vi "Force Offset Tags DAO.vi"(8 "error in (no error)":errorcluster, 11 "DAO Actions":T1) -> (0 "error out":errorcluster, 2 "Force Tags":string[](array[string]))   [LabVIEW 2009]
uses:
  Data Access Objects/Metadata/DAO Actions.ctl
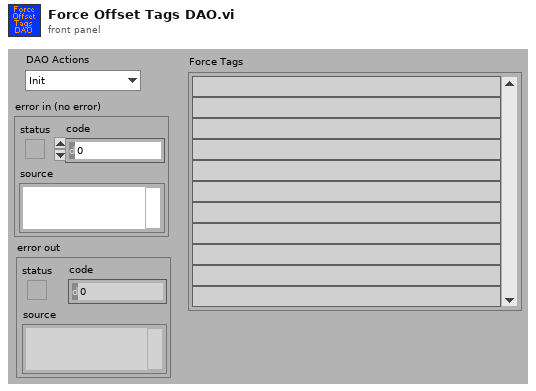
[diagram p1: front panel]
types:
  T1 = typedef "DAO Actions.ctl" = enum16{"Init", "Get", "Set"}
  T2 = typedef "Dataset Transaction Id.ctl" = cluster{"Dataset Source":T3, "Dataset Type":T4, "Hold":T5, "Volts":T5, "Tag":string}
  T3 = typedef "Dataset Source.ctl" = enum16{"LBCB 1", "LBCB 2", "Combined", "External Sensors"}
  T4 = typedef "Dataset Type.ctl" = enum16{"LVDT", "Load Cell", "Actuator Command", "Servo Error", "Displacement Command", "Displacement", "Force"}
  T5 = typedef "Yes No Button.ctl" = bool
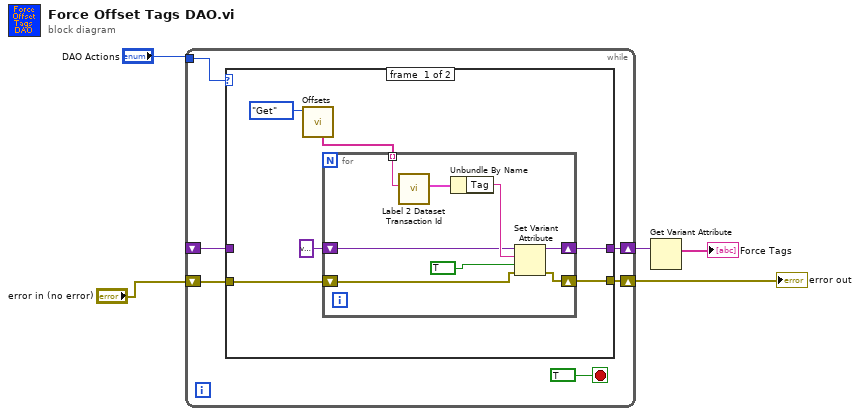
[diagram p0: block diagram]
diagram:
  n1 = while {
    tunnel: "DAO Actions" -> [w10]
    shift-right: [w9] -> w4
    shift-left: _ -> [w8]
    shift-right: [w6] -> w1
    shift-left: "error in (no error)" -> [w7]
    stop <- TRUE stop-if-true
    n2 = case shown="\"Init\", Default" w10 {
      tunnel: [w15 w27] -> w9
      tunnel: w8 -> [_ w27]
      tunnel: w7 -> [w13 w26]
      tunnel: [w12 w26] -> w6
      frame #0 {
        n3 = call "Offsets.vi"("DAO Actions"=DAO_Actions."Get") -> ("Labels"=w16:string[])  [unwired: 8 in, 2 out]
        n4 = for {
          tunnel: w16 -> [w25] mode=indexing
          shift-right: [w22] -> w15
          shift-left: variant -> [w21]
          shift-right: [w18] -> w12
          shift-left: w13 -> [w19]
          n5 = call "Label 2 Dataset Transaction Id.vi"("Label"=w25) -> ("Dataset Trans Id"=w24:T2)  [unwired: 10 in]
          n6 = Unbundle By Name(w24) -> ("Tag"=w23:string)
          n7 = Set Variant Attribute(Variant=w21, name=w23, value=TRUE, error in=w19) -> (Variant out=w22:variant, error out=w18:errorcluster)  [unwired: 1 out]
        }
      }
      frame #1 {
      }
    }
  }
  "error out" <- w1
  n8 = Get Variant Attribute(Variant=w4) -> (names=→"Force Tags":string[])  [unwired: 3 in, 3 out]
